vi "state_sep.vi"(0 "Register value":variant, 5 "MODE":u8) -> (17 "自检状态及船舱标志":string, 20 "G1陀螺脉冲数":dbl, 21 "G2陀螺脉冲数":dbl, 22 "G3陀螺脉冲数":dbl, 23 "A1加速度计脉冲数":dbl, 24 "A2加速度计脉冲数":dbl, 25 "温度":string, 26 "脉冲计数":string, 27 "A3加速度计脉冲数":dbl)   [LabVIEW 2012]
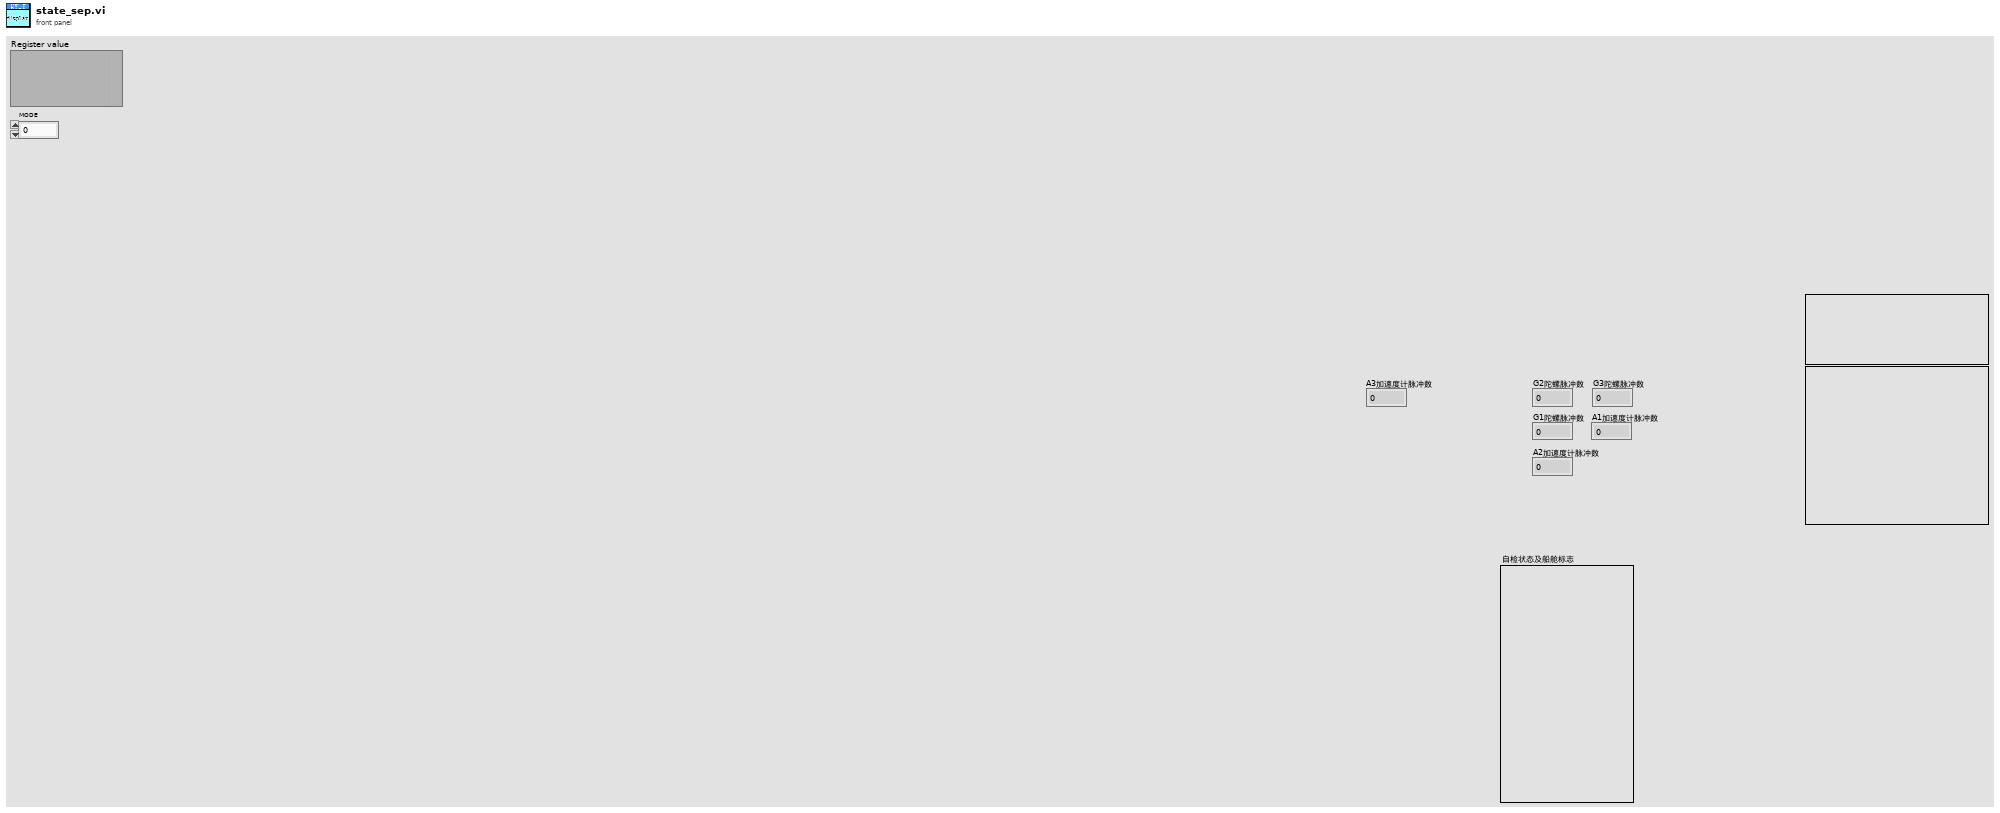
[diagram p1: front panel]
types:
  T1 = cluster{"G1陀螺脉冲数":i32, "G2陀螺脉冲数":i32, "G3陀螺脉冲数":i32, "A1加速度计脉冲数":i16, "A2加速度计脉冲数":i16, "A3加速度计脉冲数":i16, "G1陀螺自检状态":u8, "G1陀螺光路温度":i8, "G2陀螺自检状态":u8, "G2陀螺光路温度":i8, "G3陀螺自检状态":u8, "G3陀螺光路温度":i8, "A1自检状态":u8, "A1幅值":u8, "A2自检状态":u8, "A2幅值":u8, "A3自检状态":u8, "A3幅值":u8, "IF1电路温度":i8, "IF2电路温度":i8, "IF3电路温度":i8, "温控自检字":u8, "加计温度1":i16, "加计温度2":i16, "LTU状态":u8, "帧计数":u8, "G1陀螺光路温度E-2":i16, "G2陀螺光路温度E-2":i16, "G3陀螺光路温度E-2":i16, "G1陀螺电路温度E-2":i16, "G2陀螺电路温度E-2":i16, "G3陀螺电路温度E-2":i16}
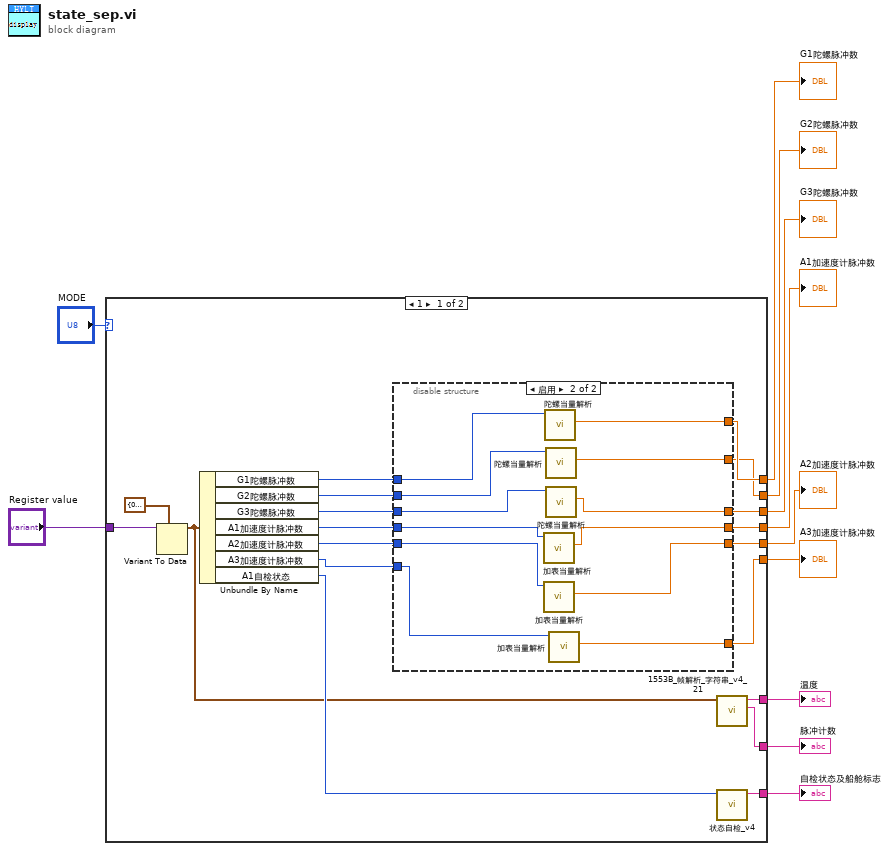
[diagram p0: block diagram]
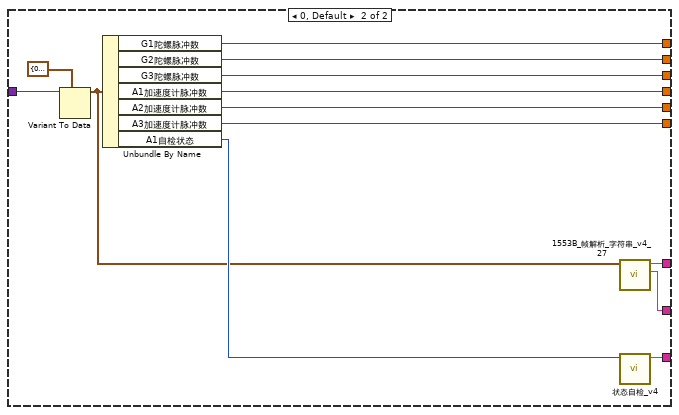
[diagram p3: hidden frame]
diagram:
  n1 = case shown="1" "MODE" {
    tunnel: "Register value" -> [w30 w55]
    tunnel: [w29 w54] -> w11
    tunnel: [w17 w53] -> w5
    tunnel: [w16 w52] -> w6
    tunnel: [w15 w51] -> w4
    tunnel: [w14 w50] -> w3
    tunnel: [w13 w49] -> w2
    tunnel: [w12 w47] -> w1
    tunnel: [w28 w48] -> w10
    tunnel: [w27 w46] -> w9
    frame 1 {
      n2 = Variant To Data(type=T1 {"G1陀螺脉冲数"=0, "G2陀螺脉冲数"=0, "G3陀螺脉冲数"=0, "A1加速度计脉冲数"=0, "A2加速度计脉冲数"=0, "A3加速度计脉冲数"=0, "G1陀螺自检状态"=0, "G1陀螺光路温度"=0, "G2陀螺自检状态"=0, "G2陀螺光路温度"=0, "G3陀螺自检状态"=0, "G3陀螺光路温度"=0, "A1自检状态"=0, "A1幅值"=0, "A2自检状态"=0, "A2幅值"=0, "A3自检状态"=0, "A3幅值"=0, "IF1电路温度"=0, "IF2电路温度"=0, "IF3电路温度"=0, "温控自检字"=0, "加计温度1"=0, "加计温度2"=0, "LTU状态"=0, "帧计数"=0, "G1陀螺光路温度E-2"=0, "G2陀螺光路温度E-2"=0, "G3陀螺光路温度E-2"=0, "G1陀螺电路温度E-2"=0, "G2陀螺电路温度E-2"=0, "G3陀螺电路温度E-2"=0} ("输入簇"), Variant=w30) -> (data=w25:T1)  [unwired: 1 in, 1 out]
      n3 = Unbundle By Name(w25) -> ("G1陀螺脉冲数"=w18:i32, "G2陀螺脉冲数"=w23:i32, "G3陀螺脉冲数"=w22:i32, "A1加速度计脉冲数"=w21:i16, "A2加速度计脉冲数"=w20:i16, "A3加速度计脉冲数"=w19:i16, "A1自检状态"=w26:u8)
      n4 = disable-structure shown="启用" {
        disable-tunnel: w18 -> [_ w42]
        disable-tunnel: w23 -> [_ w41]
        disable-tunnel: w22 -> [_ w40]
        disable-tunnel: w21 -> [_ w39]
        disable-tunnel: w20 -> [_ w38]
        disable-tunnel: w19 -> [_ w37]
        disable-tunnel: [_ w36] -> w17
        disable-tunnel: [_ w35] -> w16
        disable-tunnel: [_ w34] -> w15
        disable-tunnel: [_ w33] -> w14
        disable-tunnel: [_ w32] -> w13
        disable-tunnel: [_ w31] -> w12
        frame Disabled {
        }
        frame Enabled {
          n5 = call "加表当量解析.vi"("输入"=w39) -> ("x/y"=w33:sgl)  [unwired: 9 in, 1 out]
          n6 = call "加表当量解析.vi"("输入"=w38) -> ("x/y"=w32:sgl)  [unwired: 9 in, 1 out]
          n7 = call "陀螺当量解析.vi"("输入"=w42) -> ("x/y"=w36:sgl)  [unwired: 9 in, 1 out]
          n8 = call "陀螺当量解析.vi"("输入"=w41) -> ("x/y"=w35:sgl)  [unwired: 9 in, 1 out]
          n9 = call "陀螺当量解析.vi"("输入"=w40) -> ("x/y"=w34:sgl)  [unwired: 9 in, 1 out]
          n10 = call "加表当量解析.vi"("输入"=w37) -> ("x/y"=w31:sgl)  [unwired: 9 in, 1 out]
        }
      }
      n11 = call "1553B_帧解析_字符串_v4_21.vi"("输入簇"=w25) -> ("脉冲数"=w27:string, "温度"=w28:string)  [unwired: 9 in]
      n12 = call "状态自检_v4.vi"("陀螺自检状态字"=w26) -> ("连接的字符串"=w29:string)  [unwired: 10 in]
    }
    frame 0, Default {
      n13 = Variant To Data(type=T1 {"G1陀螺脉冲数"=0, "G2陀螺脉冲数"=0, "G3陀螺脉冲数"=0, "A1加速度计脉冲数"=0, "A2加速度计脉冲数"=0, "A3加速度计脉冲数"=0, "G1陀螺自检状态"=0, "G1陀螺光路温度"=0, "G2陀螺自检状态"=0, "G2陀螺光路温度"=0, "G3陀螺自检状态"=0, "G3陀螺光路温度"=0, "A1自检状态"=0, "A1幅值"=0, "A2自检状态"=0, "A2幅值"=0, "A3自检状态"=0, "A3幅值"=0, "IF1电路温度"=0, "IF2电路温度"=0, "IF3电路温度"=0, "温控自检字"=0, "加计温度1"=0, "加计温度2"=0, "LTU状态"=0, "帧计数"=0, "G1陀螺光路温度E-2"=0, "G2陀螺光路温度E-2"=0, "G3陀螺光路温度E-2"=0, "G1陀螺电路温度E-2"=0, "G2陀螺电路温度E-2"=0, "G3陀螺电路温度E-2"=0} ("输入簇"), Variant=w55) -> (data=w43:T1)  [unwired: 1 in, 1 out]
      n14 = Unbundle By Name(w43) -> ("G1陀螺脉冲数"=w53:i32, "G2陀螺脉冲数"=w52:i32, "G3陀螺脉冲数"=w51:i32, "A1加速度计脉冲数"=w50:i16, "A2加速度计脉冲数"=w49:i16, "A3加速度计脉冲数"=w47:i16, "A1自检状态"=w45:u8)
      n15 = call "1553B_帧解析_字符串_v4_27.vi"("输入簇"=w43) -> ("脉冲数"=w46:string, "温度"=w48:string)  [unwired: 9 in]
      n16 = call "状态自检_v4.vi"("陀螺自检状态字"=w45) -> ("连接的字符串"=w54:string)  [unwired: 10 in]
    }
  }
  "自检状态及船舱标志" <- w11
  "脉冲计数" <- w9
  "温度" <- w10
  "G2陀螺脉冲数" <- w6
  "G1陀螺脉冲数" <- w5
  "G3陀螺脉冲数" <- w4
  "A1加速度计脉冲数" <- w3
  "A2加速度计脉冲数" <- w2
  "A3加速度计脉冲数" <- w1
